vi "Calculate.vi"(8 "error in (no error)":errorcluster, 10 "X (degrees)":dbl, 11 "AngleFunction in":refnum<class "LinearInterpolation.lvclass">) -> (0 "error out":errorcluster, 2 "AngleFunction(X)":dbl, 3 "AngleFunction out":refnum<class "LinearInterpolation.lvclass">)   [LabVIEW 2012, in "LinearInterpolation.lvclass"]
doc: "Takes in saved line parameters and uses them with RetrieveValue.vi to find the value corresponding to the\ninputted angle from 0-360 degrees."
uses:
  LinearInterpolation.lvclass
  LinearInterpolation.lvclass/LinearInterpolation.ctl
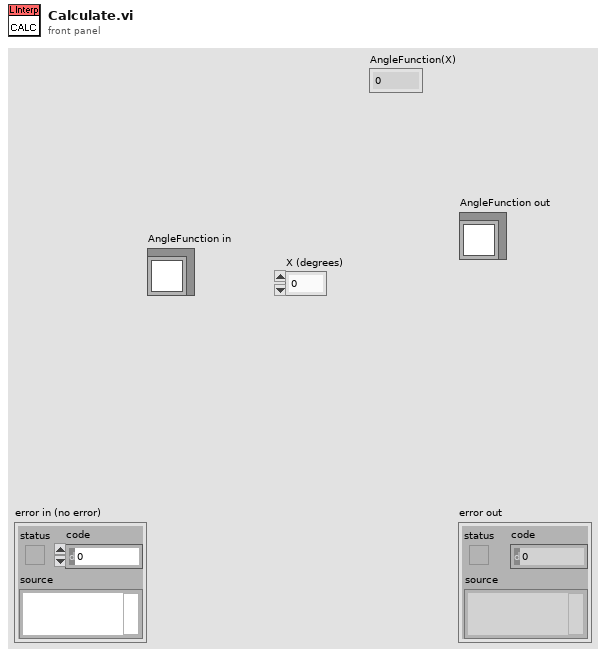
[diagram p1: front panel]
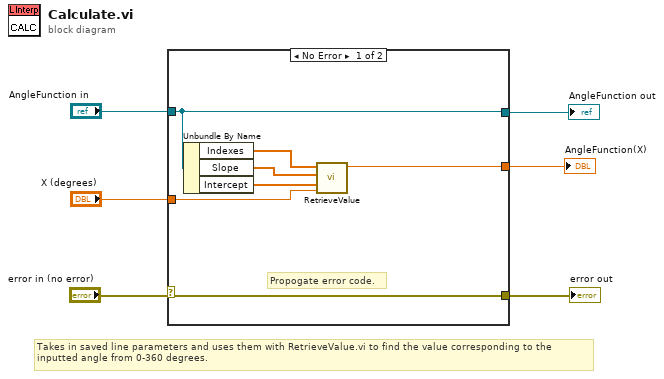
[diagram p0: block diagram]
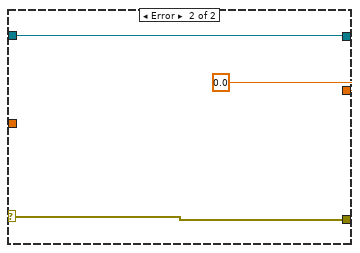
[diagram p2: hidden frame]
diagram:
  # "Takes in saved line parameters and uses them with RetrieveValue.vi to find the value corresponding to the\ninputted angle from 0-360 degrees."
  n1 = case shown="No Error" "error in (no error)" {
    selector: "error in (no error)" -> [w13 w15]
    tunnel: "AngleFunction in" -> [w12 w16]
    tunnel: "X (degrees)" -> [w8 _]
    tunnel: [w13 w15] -> w3
    tunnel: [w12 w16] -> w2
    tunnel: [w7 0.0 ("InterpolatedValue")] -> w1
    frame No Error {
      # "Propogate error code."
      n2 = Unbundle By Name(w12) -> ("Indexes"=w11:dbl[], "Slope"=w10:dbl[], "Intercept"=w9:dbl[])
      n3 = call "RetrieveValue.vi"("Desired Angle Input"=w8, "Intercept"=w9, "Slope"=w10, "Angles/Indicies"=w11) -> ("Value Output"=w7:dbl)  [unwired: 7 in]
    }
    frame Error {
    }
  }
  "error out" <- w3
  "AngleFunction out" <- w2
  "AngleFunction(X)" <- w1
